vi "Target Gen.vi"(3 "error in":errorcluster caption="error in (no error)", 4 "Sine Wave Para":T1) -> (7 "Center Coordinates":sgl[](array[numeric]), 8 "Absolute Coordinates Out":T2, 9 "Relative Coordinates Out":sgl[](array[numeric]), 10 "error out":errorcluster)   [LabVIEW 2016]
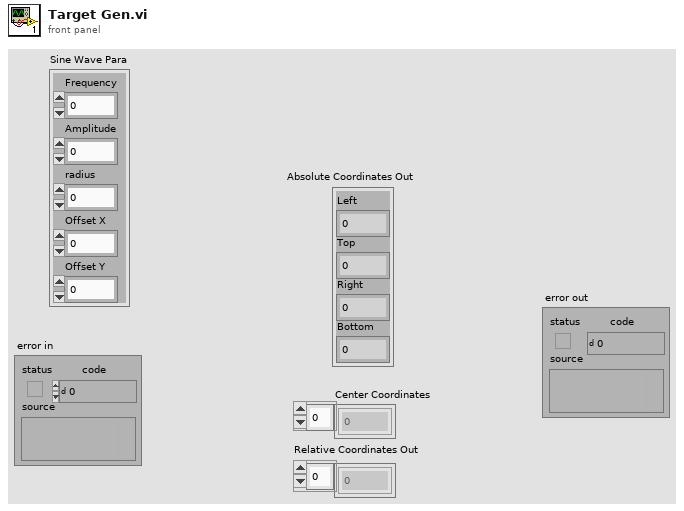
[diagram p1: front panel]
types:
  T1 = cluster{"Frequency":dbl, "Amplitude":dbl, "radius":dbl, "Offset X":dbl, "Offset Y":dbl}
  T2 = cluster{"Left":i32, "Top":i32, "Right":i32, "Bottom":i32}
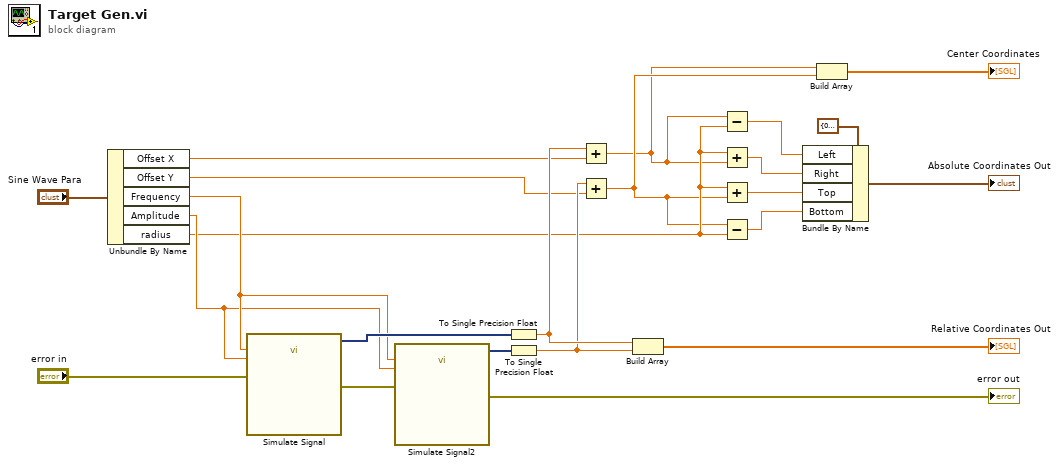
[diagram p0: block diagram]
diagram:
  n1 = Unbundle By Name("Sine Wave Para") -> ("Offset X"=w4:dbl, "Offset Y"=w5:dbl, "Frequency"=w7:dbl, "Amplitude"=w6:dbl, "radius"=w3:dbl)
  n2 = call "Simulate Signal"("Frequency"=w7, "Amplitude"=w6, "error in (no error)"="error in") -> ("Sine"=w22:dynamicdata, "error out"=w11:errorcluster)  [unwired: 11 in]
  n3 = call "Simulate Signal2"("Frequency"=w7, "Amplitude"=w6, "error in (no error)"=w11) -> ("Sine"=w21:dynamicdata, "error out"=→"error out":errorcluster)  [unwired: 11 in]
  n4 = To Single Precision Float(number=w22) -> (single precision float=w15:sgl)
  n5 = To Single Precision Float(number=w21) -> (single precision float=w14:sgl)
  n6 = Add(x=w15, y=w4) -> (x+y=w1:dbl)
  n7 = Add(x=w14, y=w5) -> (x+y=w2:dbl)
  n8 = Build Array(w15, w14) -> (→"Relative Coordinates Out":sgl[])
  n9 = Subtract(x=w1, y=w3) -> (x-y=w20:dbl)
  n10 = Add(x=w3, y=w1) -> (x+y=w18:dbl)
  n11 = Add(x=w3, y=w2) -> (x+y=w17:dbl)
  n12 = Subtract(x=w2, y=w3) -> (x-y=w19:dbl)
  n13 = Bundle By Name(cluster=T2 {"Left"=0, "Top"=0, "Right"=0, "Bottom"=0} ("Bounding Rectangle"), "Left"=w20, "Right"=w18, "Top"=w17, "Bottom"=w19) -> (→"Absolute Coordinates Out":T2)
  n14 = Build Array(w1, w2) -> (→"Center Coordinates":dbl[])
